vi "Slave Launched.vi"(8 "error in":errorcluster, 10 "SlaveID":i32) -> (0 "error out":errorcluster)   [LabVIEW 2021, in "Master.lvlib"]
doc: "This will broadcast Slaves ID launched\n_____\nCreated using DQMH Event Scripter 6.1.0.128."
uses:
  Master.lvlib
  Slave Launched Argument--cluster.ctl
  <vilib>/DQMH Consortium/Lumos API/Libraries/SDV API/SDV API.lvlib
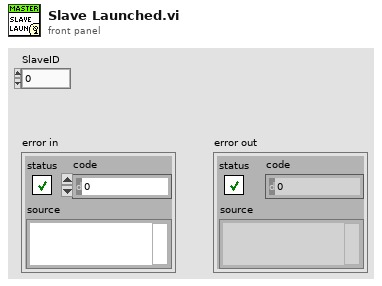
[diagram p1: front panel]
types:
  T1 = typedef "Master.lvlib/Slave Launched Argument--cluster.ctl" = cluster{"SlaveID":i32}
  T2 = typedef "Master.lvlib/Broadcast Events--cluster.ctl" = cluster{"Module Did Init":refnum<user-event>, "Status Updated":refnum<user-event>, "Error Reported":refnum<user-event>, "Module Did Stop":refnum<user-event>, "Update Module Execution Status":refnum<user-event>, "Slave Launched":refnum<user-event>}
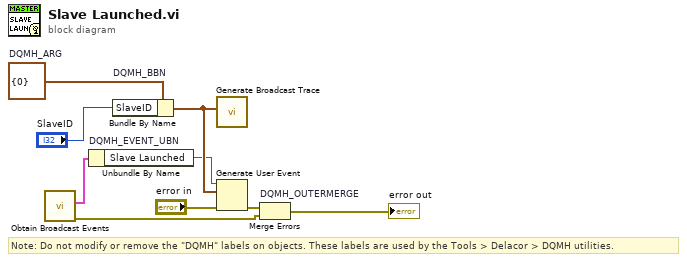
[diagram p0: block diagram]
diagram:
  w4 = T1 {"SlaveID"=0}  # DQMH_ARG
  # "Note: Do not modify or remove the \"DQMH\" labels on objects. These labels are used by the Tools > Delacor > DQMH utilities."
  n1 = call "Obtain Broadcast Events.vi"() -> ("error out"=w2:errorcluster, "Master Broadcast Events"=w1:T2)  [unwired: 10 in]
  n2 = Unbundle By Name "DQMH_EVENT_UBN"(w1) -> ("Slave Launched"=w6:refnum<user-event>)
  n3 = Bundle By Name "DQMH_BBN"(cluster=w4, "SlaveID"="SlaveID") -> (w7:T1)
  n4 = call <vilib>:"Generate Broadcast Trace.vi"("Payload"=w7) -> ()  [unwired: 10 in, 1 out]
  n5 = Generate User Event(user event=w6, event data cluster=w7, error in="error in") -> (error out=w5:errorcluster)  [unwired: 1 in, 1 out]
  n6 = Merge Errors "DQMH_OUTERMERGE"(w5, w2) -> (→"error out":errorcluster)
